vi "FindScriptPorts.vi"(1 "Input FOR VOC":u8[](array[numeric]), 2 "Test":string) -> (0 "Result Input FOR VOC":u8[](array[numeric]))   [LabVIEW 2012]
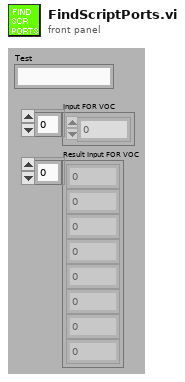
[diagram p1: front panel]
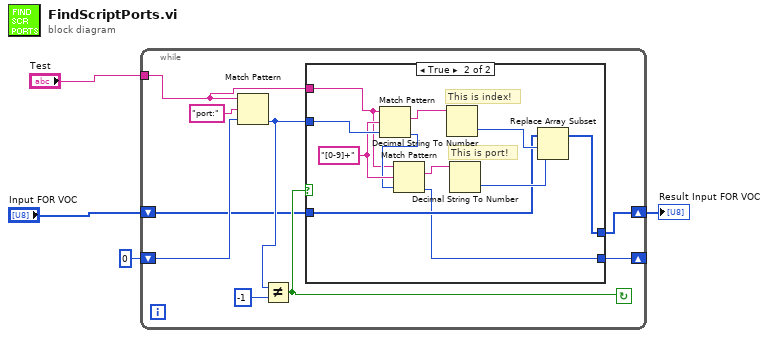
[diagram p0: block diagram]
diagram:
  n1 = while {
    shift-right: [w6] -> _
    shift-left: 0 ("offset past match") -> [w12]
    tunnel: "Test" -> [w9]
    shift-right: [w5] -> w1
    shift-left: "Input FOR VOC" -> [w7]
    stop <- w10 continue-if-true
    n2 = Match Pattern(string=w9, regular expression="port:" ("search string"), offset (0)=w12) -> (offset past match=w8:i32)  [unwired: 3 out]
    n3 = Not Equal?(x=w8, y=-1) -> (x != y?=w10:bool)
    n4 = case shown="True" w10 {
      tunnel: w9 -> [_ w23]
      tunnel: w8 -> [w15 w26]
      tunnel: w7 -> [w14 w18]
      tunnel: [w15 w17] -> w6
      tunnel: [w14 w16] -> w5
      frame False {
      }
      frame True {
        w25 = "[0-9]+" ("regular expression")
        # "This is port!"
        # "This is index!"
        n5 = Match Pattern(string=w23, regular expression=w25, offset (0)=w26) -> (match substring=w22:string, offset past match=w24:i32)  [unwired: 2 out]
        n6 = Match Pattern(string=w23, regular expression=w25, offset (0)=w24) -> (match substring=w21:string, offset past match=w17:i32)  [unwired: 2 out]
        n7 = Decimal String To Number(string=w22) -> (number=w20:i32)  [unwired: 2 in, 1 out]
        n8 = Decimal String To Number(string=w21) -> (number=w19:i32)  [unwired: 2 in, 1 out]
        n9 = Replace Array Subset(array=w18, new element=w19, index=w20) -> (w16:u8[])
      }
    }
  }
  "Result Input FOR VOC" <- w1
